vi "CalcMassSubsets.vi"(11 "Pod Coordinates":cluster{"X":dbl, "Y":dbl}[](array[cluster])) -> (3 "Mass Subsets":dbl[](array[numeric]))   [LabVIEW 2014]
uses:
  Variables/Physical data.vi
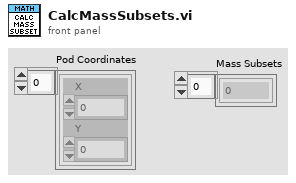
[diagram p1: front panel]
types:
  T1 = typedef "NI_Matrix.lvlib/RealMatrix.ctl" = dbl[][]
  T2 = cluster{"All Pod State Data":cluster{"Drive":cluster{"Drive Motor Output":dbl, "Wheel RPM":dbl, "Linear speed":dbl, "Linear acceleration":dbl, "Encoder Output":dbl, "Vmot":dbl, "Imot":dbl, "Torque":dbl, "Angular Momentum":dbl}, "Turret":cluster{"Turret Motor Output":dbl, "Turret Angle":dbl, "Turret velocity":dbl, "Turret acceleration":dbl, "Encoder Output":dbl, "Vmot":dbl, "Imot":dbl, "Torque":dbl, "Angular Momentum":dbl}, "Pod position (RCS)":cluster{"X":dbl, "Y":dbl, "Z":dbl}}[], "Global Robot Data":cluster{"Position Data":cluster{"Robot Position":cluster{"X":dbl, "Y":dbl, "Z":dbl}, "Robot Velocity":cluster{"X":dbl, "Y":dbl, "Z":dbl}, "Robot Acceleration":cluster{"X":dbl, "Y":dbl, "Z":dbl}}, "Rotation Data":cluster{"Angular Position":cluster{"X":dbl, "Y":dbl, "Z":dbl}, "Angular Velocity":cluster{"X":dbl, "Y":dbl, "Z":dbl}, "Angular Acceleration":cluster{"X":dbl, "Y":dbl, "Z":dbl}}}, "Inertial Characteristics":cluster{"Center of Mass (RCS)":cluster{"X":dbl, "Y":dbl, "Z":dbl}, "Mass Elements":cluster{"X":dbl, "Y":dbl, "Z":dbl, "Mass":dbl, "Name":string}[], "Center of Rotation (RCS)":cluster{"X":dbl, "Y":dbl, "Z":dbl}, "Tensor of Inertia":T1}}
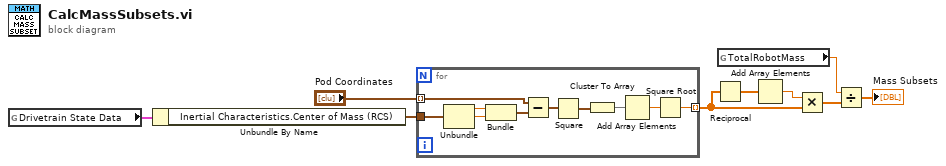
[diagram p0: block diagram]
diagram:
  n1 = global read "Physical data.vi" "Drivetrain State Data"() -> (w9:T2)
  n2 = Unbundle By Name(w9) -> ("Inertial Characteristics.Center of Mass (RCS)"=w8:cluster{"X":dbl, "Y":dbl, "Z":dbl})
  n3 = for {
    tunnel: w8 -> [w13]
    tunnel: "Pod Coordinates" -> [w19] mode=indexing
    tunnel: [w14] -> w4 mode=indexing
    n4 = Unbundle(w13) -> ("X"=w12:dbl, "Y"=w11:dbl)  [unwired: 1 out]
    n5 = Bundle("X"=w12, "Y"=w11) -> (w10:cluster{"X":dbl, "Y":dbl})  [unwired: 1 in]
    n6 = Subtract(x=w19, y=w10) -> (x-y=w18:cluster{"X":dbl, "Y":dbl})
    n7 = Square(x=w18) -> (x^2=w17:cluster{"X":dbl, "Y":dbl})
    n8 = Cluster To Array(cluster=w17) -> (array=w16:dbl[])
    n9 = Add Array Elements(numeric array=w16) -> (sum=w15:dbl)
    n10 = Square Root(x=w15) -> (sqrt(x)=w14:dbl)
  }
  n11 = Reciprocal(x=w4) -> (1/x=w6:dbl[])
  n12 = global read "Physical data.vi" "TotalRobotMass"() -> (w3:dbl)
  n13 = Add Array Elements(numeric array=w6) -> (sum=w5:dbl)
  n14 = Multiply(x=w5, y=w4) -> (x*y=w2:dbl[])
  n15 = Divide(x=w3, y=w2) -> (x/y=→"Mass Subsets":dbl[])
